vi "MH_SetHistoLen.vi"(8 "error in (no error)":errorcluster, 10 "lencode":i32, 11 "devidx":i32) -> (0 "error out":errorcluster, 2 "actuallen":i32, 3 "return type":i32)   [LabVIEW 2019]
uses:
  <userlib>/MultiHarp150/MH_DllPath_global.vi
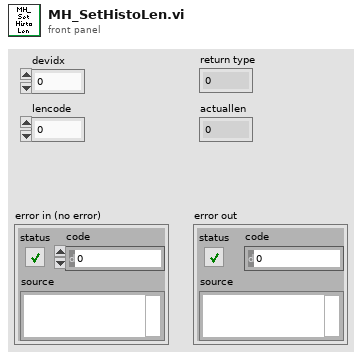
[diagram p1: front panel]
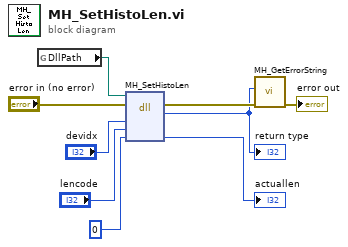
[diagram p0: block diagram]
diagram:
  n1 = global read "MH_DllPath_global.vi" "DllPath"() -> (w8:path)
  n2 = dll-call lib="MHLib64.dll" fn="MH_SetHistoLen"(path in=w8, error in="error in (no error)", "devidx"="devidx", "lencode"="lencode", "actuallen"=0 ("ctcstatus")) -> (error out=w6:errorcluster, "return type"=w5:i32, "actuallen"=→"actuallen":i32)  [unwired: 3 in, 1 out]
  "return type" <- w5
  n3 = call <userlib>:"MH_GetErrorString.vi"("error in (no error)"=w6, "code"=w5) -> ("error out"=→"error out":errorcluster)  [unwired: 7 in, 2 out]
